vi "NewBoard Runtime.vi"(8 "error in (no error)":errorcluster, 10 "Capno Data In":T2={"Port"="", "Source"=0, "Active"=FALSE, "Baro Pressure"=760, "SerialRxBuffer"="", "Raw CO2 (Torr)"=5.0, "bytes read"=5, "Status"=[], "Status Message"=enum.""} {"Status" format="%x"; "Raw CO2 (Torr)" format="%.2f"; "Baro Pressure" min=400 max=800; "Source" items=["None", "TidalWave", "LoFlow / Canary", "Capnogard"]}, 11 "reference":refnum<visa-resource-name>) -> (0 "Error Out":errorcluster, 1 "RawBytesRead":string, 2 "Capno Data Out":T2={"Port"="", "Source"=0, "Active"=FALSE, "Baro Pressure"=760, "SerialRxBuffer"="", "Raw CO2 (Torr)"=5.0, "bytes read"=5, "Status"=[], "Status Message"=enum.""} {"Status" format="%x"; "Raw CO2 (Torr)" format="%.2f"; "Baro Pressure" min=400 max=800; "Source" items=["None", "TidalWave", "LoFlow / Canary", "Capnogard"]}, 3 "Serial Port Out":T4={"termination char"=10, "End read on termination character?"=TRUE, "Enabled?"=FALSE, "VISA resource name"="COM7", "baud rate"=9600, "data bits"=8, "parity"=enum."None", "stop bits"=10, "flow control"=0, "timeout (ms)"=10000, "Input buffer size"=4096, "End write on termination character?"=FALSE, "XON Char"=17, "XOFF Char"=19} {"XOFF Char" format="%.0x"; "XON Char" format="%.0x"; "flow control" items=["None"=0, "XON/XOFF"=1, "RTS/CTS"=2, "DTR/DSR"=4]; "stop bits" items=["1.0"=10, "1.5"=15, "2.0"=20]; "baud rate" items=["1.0"=10, "1.5"=15, "2.0"=20]; "termination char" format="%.0x"})   [LabVIEW 2014]
uses:
  Libraries/Controls/Serial Visa Control.ctl
  Libraries/Controls/Aux CO2 Diags.ctl
  Libraries/Controls/Aux CO2 Selector.ctl
panel:
  out "SerialRxBuffer":string
  out "Prioritized Status":u8=100
  out "Status Message":T1(ring)
  out "DPI's":u8[][](array[numeric]) format="%x"
  out "length":i32
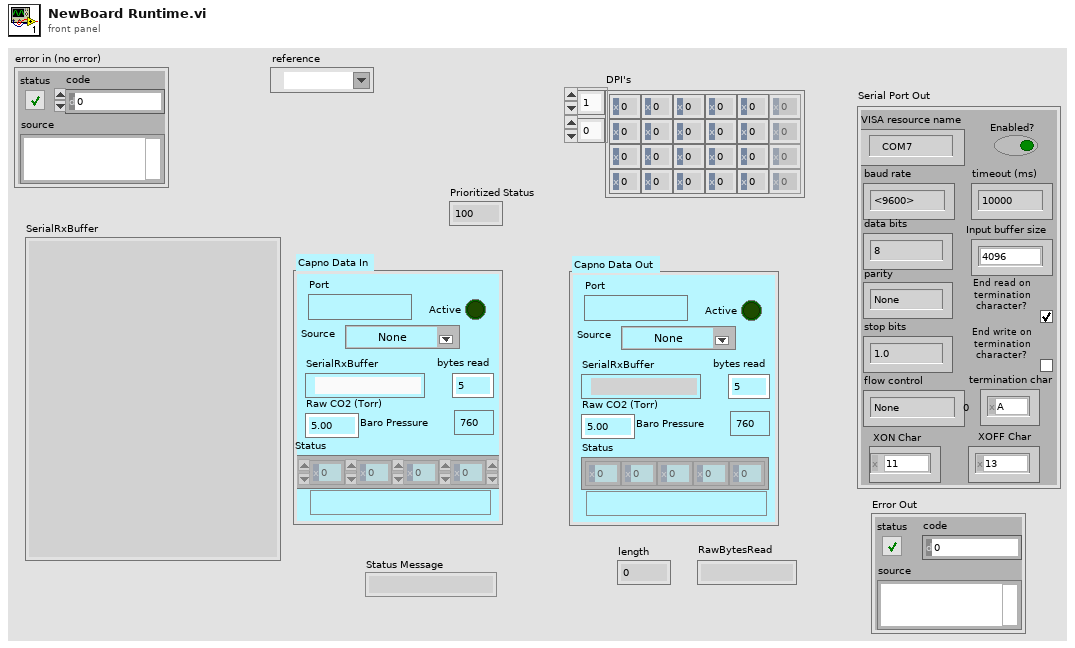
[diagram p1: front panel]
types:
  T1 = enum16{"", "Sensor Over Temp", "Sensor Faulty", "Set BaroP", "Capno in Sleep Mode", "Zero In Progress", "Sensor Warm Up", "Zero Required", "CO2 Out Of Range", "Check Airway Adapter", "Check Sampling Line", "LoFlo Not Connected"}
  T2 = typedef "Aux CO2 Diags.ctl" = cluster{"Port":refnum<visa-resource-name>, "Source":T3, "Active":bool, "Baro Pressure":u16, "SerialRxBuffer":string, "Raw CO2 (Torr)":sgl, "bytes read":i16, "Status":u8[], "Status Message":enum16{"", "Sensor Over Temp", "Sensor Faulty", "Set BaroP", "Capno in Sleep Mode", "Zero In Progress", "Sensor Warm Up", "Check Sampling Line", "Zero Required", "CO2 Out Of Range", "Check Airway Adapter", "LoFlo Not Connected"}}
  T3 = typedef "Aux CO2 Selector.ctl" = u16
  T4 = typedef "Serial Visa Control.ctl" = cluster{"termination char":u8, "End read on termination character?":bool, "Enabled?":bool, "VISA resource name":refnum<visa-resource-name>, "baud rate":u32, "data bits":u16, "parity":enum16{"None", "Odd", "Even", "Mark", "Space"}, "stop bits":u16, "flow control":u16, "timeout (ms)":u32, "Input buffer size":u32, "End write on termination character?":bool, "XON Char":u8, "XOFF Char":u8}
  T5 = enum16{"", "Sensor Over Temp", "Sensor Faulty", "Set BaroP", "Capno in Sleep Mode", "Zero In Progress", "Sensor Warm Up", "Check Sampling Line", "Zero Required", "CO2 Out Of Range", "Check Airway Adapter", "LoFlo Not Connected"}
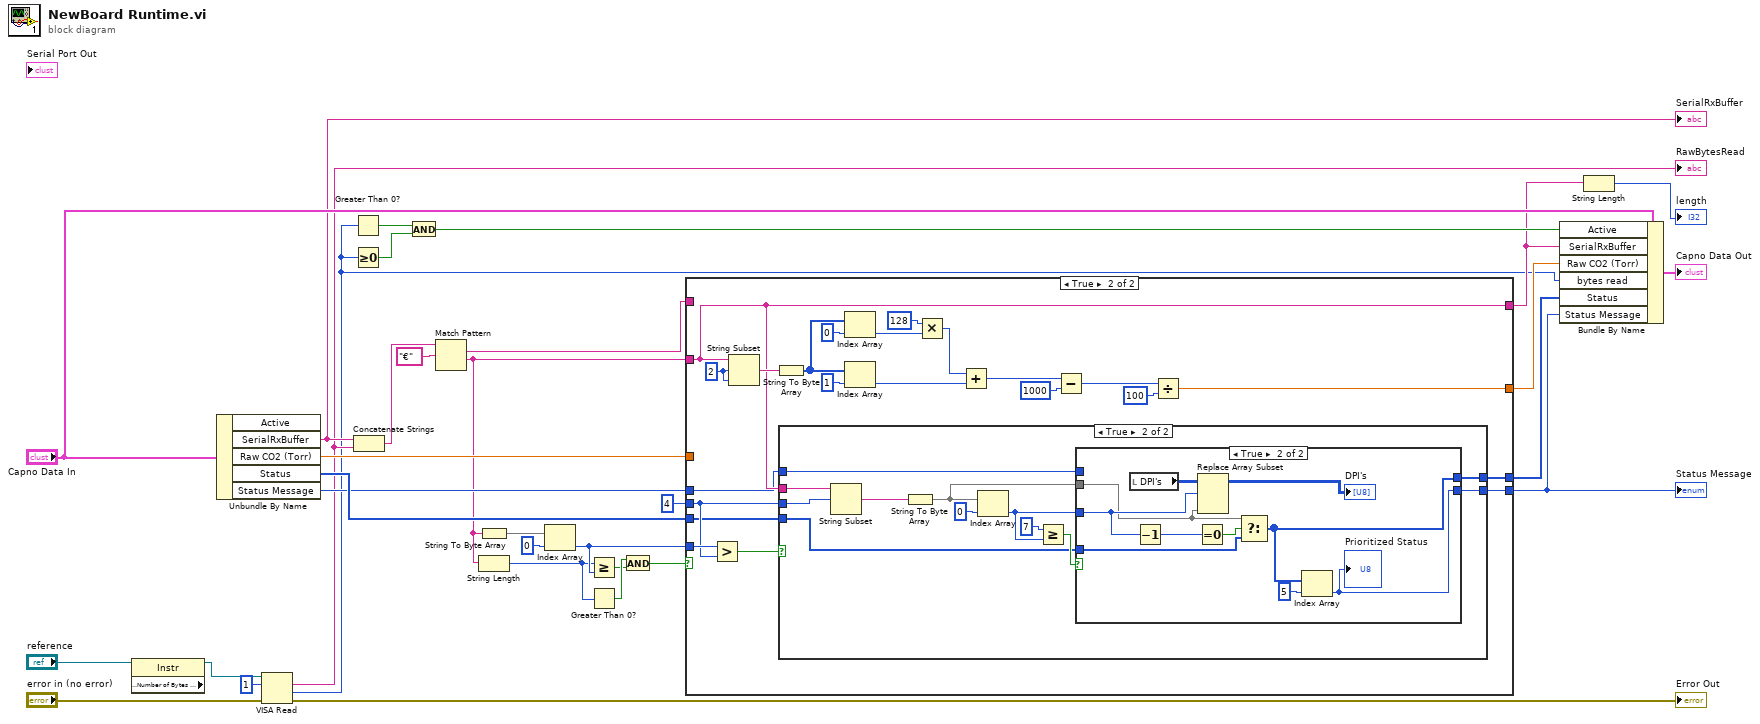
[diagram p0: block diagram]
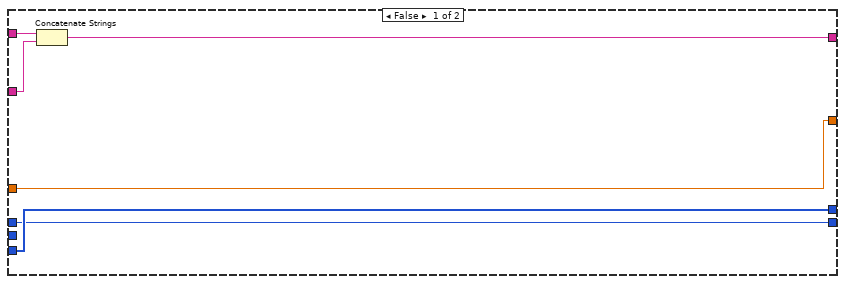
[diagram p2: hidden frame]
diagram:
  n1 = property class="Instr" props=["Serial Settings:Number of Bytes at Serial Port"](reference="reference") -> (reference out=w19:refnum<visa-resource-name>)  [unwired: 1 in, 2 out]
  n2 = Unbundle By Name("Capno Data In") -> ("SerialRxBuffer"=w28:string, "Raw CO2 (Torr)"=w29:sgl, "Status"=w25:u8[], "Status Message"=w24:T5)  [unwired: 1 out]
  "SerialRxBuffer" <- w28
  n3 = VISA Read(VISA resource name=w19, byte count=u32 1, error in (no error)="error in (no error)") -> (read buffer=w17:string, return count=w15:u32, error out=→"Error Out":errorcluster)  [unwired: 1 out]
  "RawBytesRead" <- w17
  n4 = Greater Than 0?(x=w15) -> (x > 0?=w22:bool)
  n5 = Greater Or Equal To 0?(x=w15) -> (x >= 0?=w23:bool)
  n6 = Concatenate Strings(w28, w17) -> (w13:string)
  n7 = And(x=w22, y=w23) -> (x .and. y?=w33:bool)
  n8 = Match Pattern(string=w13, regular expression="€" ("format string")) -> (match substring=w12:string, after substring=w8:string)  [unwired: 1 in, 2 out]
  n9 = String To Byte Array(string=w8) -> (unsigned byte array=w10:u8[])
  n10 = String Length(string=w8) -> (length=w5:i32)
  n11 = Index Array(array=w10, index=0) -> (element=w6:u8)
  n12 = Greater Or Equal?(x=w5, y=w6) -> (x >= y?=w3:bool)
  n13 = Greater Than 0?(x=w5) -> (x > 0?=w4:bool)
  n14 = And(x=w4, y=w3) -> (x .and. y?=w2:bool)
  n15 = case shown="True" w2 {
    tunnel: w8 -> [w38 w47]
    tunnel: w12 -> [w39 _]
    tunnel: [w37 w47] -> w27
    tunnel: [w36 w48] -> w32
    tunnel: w29 -> [w36 _]
    tunnel: 4 -> [_ w44]
    tunnel: w6 -> [_ w45]
    tunnel: w25 -> [w35 w43]
    tunnel: [w35 w42] -> w21
    tunnel: w24 -> [w34 w41]
    tunnel: [w34 w40] -> w20
    frame False {
      n16 = Concatenate Strings(w39, w38) -> (w37:string)
    }
    frame True {
      w61 = 2 ("length (rest)")
      n17 = Greater?(x=w45, y=w44) -> (0:w46:bool)
      n18 = String Subset(string=w47, offset (0)=w61, length (rest)=w61) -> (substring=w60:string)
      n19 = String To Byte Array(string=w60) -> (unsigned byte array=w57:u8[])
      n20 = case shown="True" w46 {
        tunnel: w47 -> [_ w75]
        tunnel: w44 -> [_ w68]
        tunnel: w43 -> [w63 w67]
        tunnel: [w63 w66] -> w42
        tunnel: w41 -> [w62 w65]
        tunnel: [w62 w64] -> w40
        frame False {
        }
        frame True {
          n21 = String Subset(string=w75, offset (0)=w68) -> (substring=w73:string)  [unwired: 1 in]
          n22 = String To Byte Array(string=w73) -> (unsigned byte array=w69:u8[])
          n23 = Index Array(array=w69, index=0) -> (element=w70:u8)
          n24 = Greater Or Equal?(x=7, y=w70) -> (x >= y?=w71:bool)
          n25 = case shown="True" w71 {
            tunnel: w70 -> [_ w85]
            tunnel: w69 -> [_ w82]
            tunnel: w67 -> [w77 w81]
            tunnel: [w77 w79] -> w66
            tunnel: w65 -> [w76 _]
            tunnel: [w76 w78] -> w64
            frame False {
            }
            frame True {
              n26 = local read "DPI's"() -> (w86:u8[][])
              n27 = Decrement(x=w85) -> (x-1=w84:u8)
              n28 = Equal To 0?(x=w84) -> (x = 0?=w83:bool)
              n29 = Replace Array Subset(array=w86, new element=w82, index (row)=w85) -> (→"DPI's":u8[][])  [unwired: 1 in]
              n30 = Select(t=w82, s=w83, f=w81) -> (s? t:f=w79:u8[])
              n31 = Index Array(array=w79, index=5) -> (element=w78:u8)
              "Prioritized Status" <- w78
            }
          }
        }
      }
      n32 = Index Array(array=w57, index=0) -> (element=w56:u8)
      n33 = Index Array(array=w57, index=1) -> (element=w53:u8)
      n34 = Multiply(x=128, y=w56) -> (x*y=w54:i32)
      n35 = Add(x=w54, y=w53) -> (x+y=w52:i32)
      n36 = Subtract(x=w52, y=1000) -> (x-y=w50:i32)
      n37 = Divide(x=w50, y=100) -> (x/y=w48:dbl)
    }
  }
  "Status Message" <- w20
  n38 = Bundle By Name(cluster="Capno Data In", "Active"=w33, "SerialRxBuffer"=w27, "Raw CO2 (Torr)"=w32, "bytes read"=w15, "Status"=w21, "Status Message"=w20) -> (→"Capno Data Out":T2)
  n39 = String Length(string=w27) -> (length=→"length":i32)
